vi "QuantizeFloat32_exc.vi"(4 "exception":T1 {"mantissa" format="%08x"}, 5 "invalid":bool, 7 "sticky bit":bool, 8 "underflow in":bool, 10 "float in":T1 {"mantissa" format="%08x"}) -> (1 "underflow":bool, 2 "overflow":bool, 3 "float out":T1 {"mantissa" format="%08x"})   [LabVIEW 2011]
uses:
  FPGA SGL.ctl
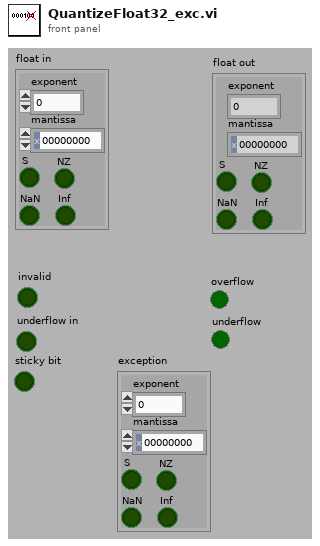
[diagram p1: front panel]
types:
  T1 = typedef "FPGA SGL.ctl" = cluster{"exponent":u8, "mantissa":u32, "S":bool, "NZ":bool, "NaN":bool, "Inf":bool}
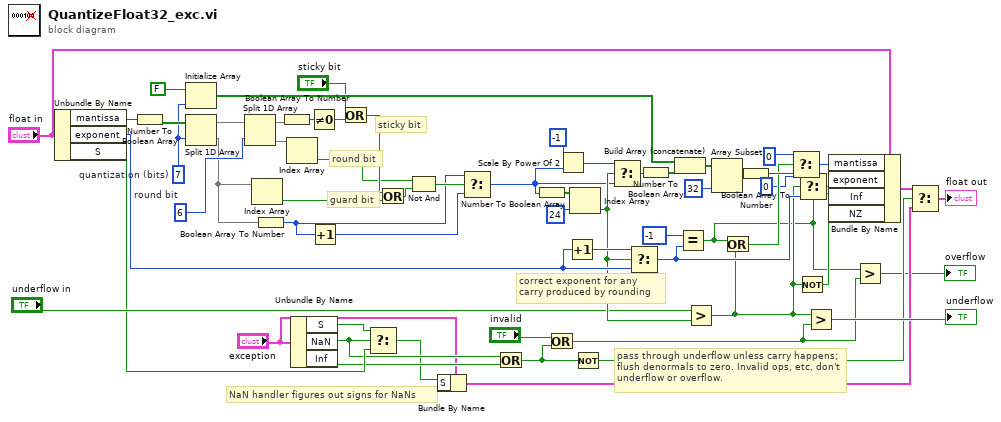
[diagram p0: block diagram]
diagram:
  w48 = 6  # round bit
  w49 = i8 7  # quantization (bits)
  # "NaN handler figures out signs for NaNs"
  # "pass through underflow unless carry happens;\nflush denormals to zero. Invalid ops, etc, don't underflow or overflow."
  # "correct exponent for any carry produced by rounding"
  # "guard bit"
  # "round bit"
  # "sticky bit"
  n1 = Unbundle By Name("float in") -> ("mantissa"=w60:u32, "exponent"=w38:u8, "S"=w23:bool)
  n2 = Number To Boolean Array(number=w60) -> (Boolean array=w59:bool[])
  n3 = Initialize Array(FALSE, w49) -> (w53:bool[])
  n4 = Split 1D Array(array=w59, index=w49) -> (first subarray=w58:bool[], second subarray=w37:bool[])
  n5 = Split 1D Array(array=w58, index=w48) -> (first subarray=w57:bool[], second subarray=w55:bool[])
  n6 = Index Array(array=w37) -> (element=w7:bool)  [unwired: 1 in]
  n7 = Boolean Array To Number(Boolean array=w37) -> (number=w3:u32)
  n8 = Boolean Array To Number(Boolean array=w57) -> (number=w56:u8)
  n9 = Index Array(array=w55) -> (element=w5:bool)  [unwired: 1 in]
  n10 = Unbundle By Name("exception") -> ("S"=w22:bool, "NaN"=w21:bool, "Inf"=w20:bool)
  n11 = Not Equal To 0?(x=w56) -> (x != 0?=w47:bool)
  n12 = Increment(x=w3) -> (x+1=w2:u32)
  n13 = Or(x="sticky bit", y=w47) -> (x .or. y?=w6:bool)
  n14 = Select(t=w22, s=w21, f=w23) -> (s? t:f=w17:bool)
  n15 = Or(x=w6, y=w7) -> (x .or. y?=w8:bool)
  n16 = Not And(1:w8, 2:w5) -> (0:w4:bool)
  n17 = Bundle By Name(cluster="exception", "S"=w17) -> (w16:T1)
  n18 = Select(t=w3, s=w4, f=w2) -> (s? t:f=w1:u32)
  n19 = Or(x=w21, y=w20) -> (x .or. y?=w12:bool)
  n20 = Number To Boolean Array(number=w1) -> (Boolean array=w45:bool[])
  n21 = Or(x="invalid", y=w12) -> (x .or. y?=w11:bool)
  n22 = Scale By Power Of 2(n=-1, x=w1) -> (x*2^n=w42:u32)
  n23 = Increment(x=w38) -> (x+1=w39:u8)
  n24 = Index Array(array=w45, index=24) -> (element=w36:bool)
  n25 = Not(x=w12) -> (.not. x?=w14:bool)
  n26 = Select(t=w42, s=w36, f=w1) -> (s? t:f=w41:u32)
  n27 = Select(t=w39, s=w36, f=w38) -> (s? t:f=w28:u8)
  n28 = Number To Boolean Array(number=w41) -> (Boolean array=w40:bool[])
  n29 = Build Array (concatenate)(w53, w40) -> (w51:bool[])
  n30 = Equal?(x=i8 -1, y=w28) -> (x = y?=w10:bool)
  n31 = Greater?(x="underflow in", y=w36) -> (0:w25:bool)
  n32 = Array Subset(array=w51, length=32) -> (w52:bool[])  [unwired: 1 in]
  n33 = Or(x=w10, y=w25) -> (x .or. y?=w30:bool)
  n34 = Boolean Array To Number(Boolean array=w52) -> (number=w34:u32)
  n35 = Select(t=u32 0, s=w30, f=w34) -> (s? t:f=w33:u32)
  n36 = Not(x=w25) -> (.not. x?=w31:bool)
  n37 = Select(t=i8 0, s=w25, f=w28) -> (s? t:f=w27:u8)
  n38 = Greater?(x=w25, y=w11) -> (0:→"underflow":bool)
  n39 = Bundle By Name(cluster="float in", "mantissa"=w33, "exponent"=w27, "Inf"=w10, "NZ"=w31) -> (w19:T1)
  n40 = Greater?(x=w10, y=w11) -> (0:→"overflow":bool)
  n41 = Select(t=w19, s=w14, f=w16) -> (s? t:f=→"float out":T1)
